vi "Read Config.vi"(8 "error in (no error)":errorcluster, 11 "Control-Client in":refnum<class "Control-Client.lvclass">) -> (0 "error out":errorcluster, 2 "Config.lvclass":refnum<class "Config.lvclass">, 3 "Control-Client out":refnum<class "Control-Client.lvclass">)   [LabVIEW 2015]
uses:
  Control-Client.lvclass
  Config/Config.lvclass
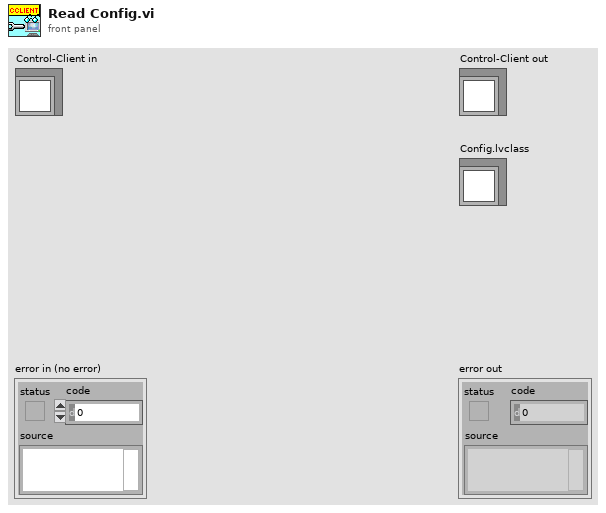
[diagram p1: front panel]
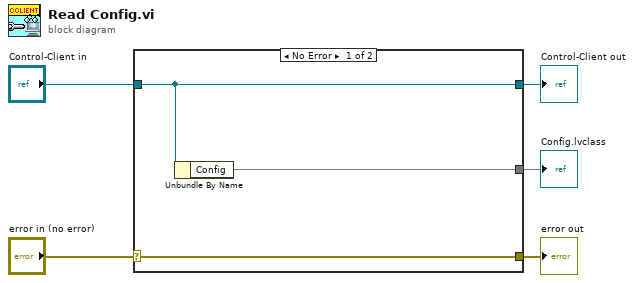
[diagram p0: block diagram]
diagram:
  n1 = case shown="No Error" "error in (no error)" {
    selector: "error in (no error)" -> [w8 w9]
    tunnel: [w8 w9] -> w4
    tunnel: [w7 w10] -> w2
    tunnel: "Control-Client in" -> [w7 w10]
    tunnel: [w6 _] -> w1
    frame No Error {
      n2 = Unbundle By Name(w7) -> ("Config"=w6)
    }
    frame Error {
    }
  }
  "error out" <- w4
  "Control-Client out" <- w2
  "Config.lvclass" <- w1
